vi "enqueueAll.vi"(8 "Waypoint Queue":refnum<queue>, 11 "Waypoint Array":refnum<class "Waypoint.lvclass">[](array[class])) -> (3 "Waypoint Queue Out":refnum<queue>)   [LabVIEW 2013]
doc: "Takes an array of elements and add all to the queue, starting with E0 and ending with En"
uses:
  Logic/Classes/Waypoint/Waypoint.lvclass
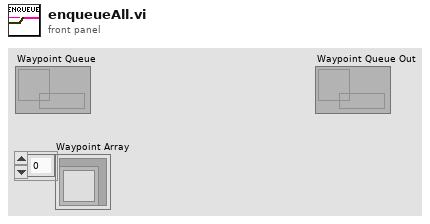
[diagram p1: front panel]
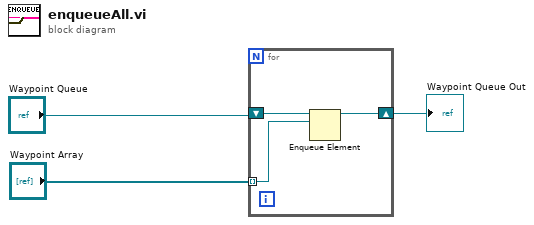
[diagram p0: block diagram]
diagram:
  n1 = for {
    shift-right: [w6] -> w3
    shift-left: "Waypoint Queue" -> [w5]
    tunnel: "Waypoint Array" -> [w4] mode=indexing
    n2 = Enqueue Element(queue=w5, element=w4) -> (queue out=w6:refnum<queue>)  [unwired: 2 in, 2 out]
  }
  "Waypoint Queue Out" <- w3
